vi "MenuActive(Data).vi"(8 "error in":errorcluster caption="错误输入（无错误）", 10 "Menu Reference in":refnum<k9>, 11 "PanelDataNode in":refnum<class "PanelDataNode.lvclass"> caption="DNL_LabVIEW Object in") -> (0 "error out":errorcluster caption="错误输出", 2 "menu reference out":refnum<k9>, 3 "PanelDataNode out":refnum<class "PanelDataNode.lvclass"> caption="DNL_LabVIEW Object out")   [LabVIEW 2016, in "PanelDataNode.lvclass"]
uses:
  PanelDataNode.lvclass
  PanelDataNode.lvclass/PanelDataNode.ctl
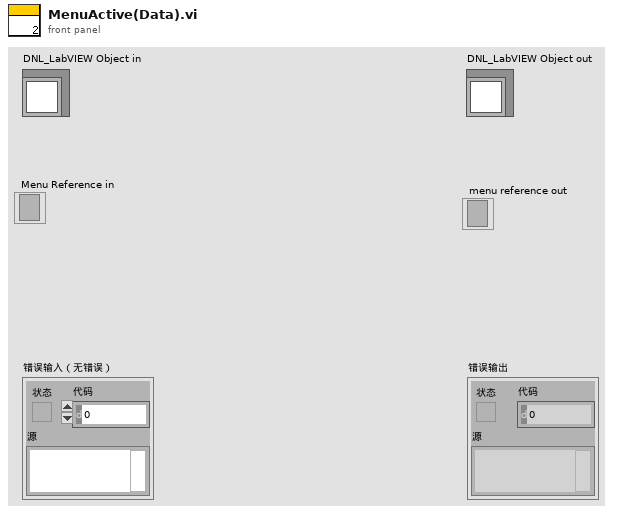
[diagram p1: front panel]
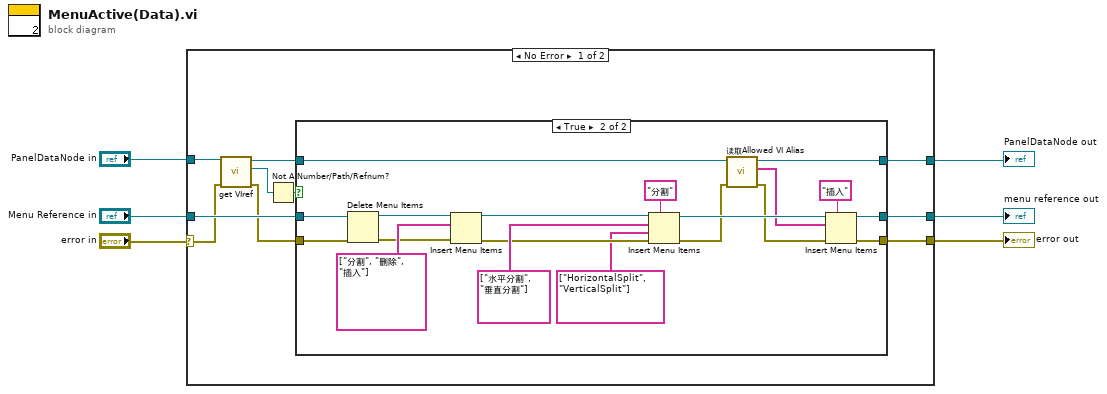
[diagram p0: block diagram]
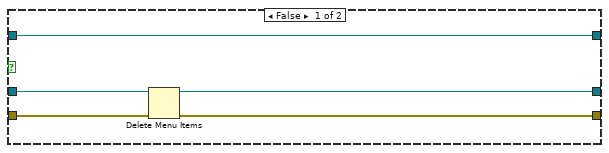
[diagram p2: hidden frame]
diagram:
  n1 = case shown="No Error" "error in" {
    selector: "error in" -> [w8 w43]
    tunnel: [w15 w42] -> w5
    tunnel: [w16 w43] -> w4
    tunnel: "PanelDataNode in" -> [w12 w42]
    tunnel: "Menu Reference in" -> [w11 w41]
    tunnel: [w10 w41] -> w1
    frame No Error {
      n2 = call "get VIref.vi"("error in (no error)"=w8, "PanelDataNode输入"=w12) -> ("error out"=w7:errorcluster, "VI*"=w9:refnum<vi>, "PanelDataNode输出"=w14:refnum<class "PanelDataNode.lvclass">)  [unwired: 7 in]
      n3 = Not A Number/Path/Refnum?(number/path/refnum=w9) -> (NaN/Path/Refnum?=w13:bool)
      n4 = case shown="True" w13 {
        tunnel: [w18 w31] -> w16
        tunnel: w14 -> [w21 w29]
        tunnel: [w21 w27] -> w15
        tunnel: w7 -> [w19 w26]
        tunnel: w11 -> [w20 w25]
        tunnel: [w17 w24] -> w10
        frame False {
          n5 = Delete Menu Items(6:w19, 9:w20) -> (0:w18:errorcluster, 3:w17:refnum<k9>)  [unwired: 2 in]
        }
        frame True {
          n6 = Delete Menu Items(6:w26, 9:w25) -> (0:w35:errorcluster, 3:w40:refnum<k9>)  [unwired: 2 in]
          n7 = Insert Menu Items(6:w35, 8:string[] ["分割", "删除", "插入"] ("项名称"), 9:w40) -> (0:w34:errorcluster, 3:w38:refnum<k9>)  [unwired: 3 in, 1 out]
          n8 = Insert Menu Items(5:"分割" ("菜单标识符"), 6:w34, 7:string[] ["HorizontalSplit", "VerticalSplit"] ("项标识符"), 8:string[] ["水平分割", "垂直分割"] ("项名称"), 9:w38) -> (0:w23:errorcluster, 3:w32:refnum<k9>)  [unwired: 1 in, 1 out]
          n9 = call "读取Allowed VI Alias.vi"("error in (no error)"=w23, "PanelDataNode输入"=w29) -> ("error out"=w22:errorcluster, "Allowed VI Alias"=w28:string[], "PanelDataNode输出"=w27:refnum<class "PanelDataNode.lvclass">)  [unwired: 7 in]
          n10 = Insert Menu Items(5:"插入" ("菜单标识符"), 6:w22, 8:w28, 9:w32) -> (0:w31:errorcluster, 3:w24:refnum<k9>)  [unwired: 2 in, 1 out]
        }
      }
    }
    frame Error {
    }
  }
  "error out" <- w4
  "PanelDataNode out" <- w5
  "menu reference out" <- w1
